vi "ADS1015 Read All.vi"(8 "error in (no error)":errorcluster, 9 "ADS1015 Config Options":T1={"I2C"={"Slave Address"=72, "Channel"=1}, "ADC"={"Channel"=4, "Expected Range (Programmable Gain Amplifier)"=0, "Sampling Mode"=1, "Sampling Rate"=4, "Comparator Mode"=1, "Comparator Polarity"=1, "Latching Comparator"=1, "Comparator Queue & Disable"=3}} {"ADC"."Comparator Queue & Disable" items=["Assert after one conversion", "Assert after two conversions", "Assert after four conversions", "Comparator disabled"]; "ADC"."Latching Comparator" items=["Non-latching", "Latching"]; "ADC"."Comparator Polarity" items=["Active Low", "Active High"]; "ADC"."Comparator Mode" items=["Traditional Comparator w/ hysteresis", "Window Comparator"]; "ADC"."Sampling Rate" items=["128SPS", "250SPS", "490SPS", "920SPS", "1600SPS", "2400SPS", "3300SPS"]; "ADC"."Sampling Mode" items=["Continuous Conversion", "Single-shot (Low Power)"]; "ADC"."Expected Range (Programmable Gain Amplifier)" items=["+/-6.144V", "+/-4.096V", "+/-2.048V", "+/-1.024V", "+/-0.512V", "+/-0.256V"]; "ADC"."Channel" items=["Differential: Ch 0&1", "Differential: Ch 0&3", "Differential: Ch 1&3", "Differential: Ch 2&3", "Single Ended: Ch 0", "Single Ended: Ch 1", "Single Ended: Ch 2", "Single Ended: Ch 3"]; "I2C"."Slave Address" format="%.0x"}, 11 "LINX Resource in":T2) -> (0 "error out":errorcluster, 2 "Voltages":dbl[](array[numeric]) format="%.3f V", 3 "LINX Resource":T2, 4 "Resolutions":dbl[](array[numeric]) format="%.3f V")   [LabVIEW 2017]
uses:
  <vilib>/MakerHub/LINX/Private/Type Defs/Platform.ctl
  <vilib>/MakerHub/LINX/Private/Type Defs/Interface.ctl
  <vilib>/MakerHub/LINX/Private/Device/Type Defs/TCP Config.ctl
  <vilib>/MakerHub/LINX/Private/Device/Type Defs/Channels.ctl
  <vilib>/MakerHub/LINX/Private/Device/Type Defs/LINX Device Config.ctl
  <vilib>/MakerHub/LINX/Private/Type Defs/LINX Ref.ctl
  ADS1015 Config Options.ctl
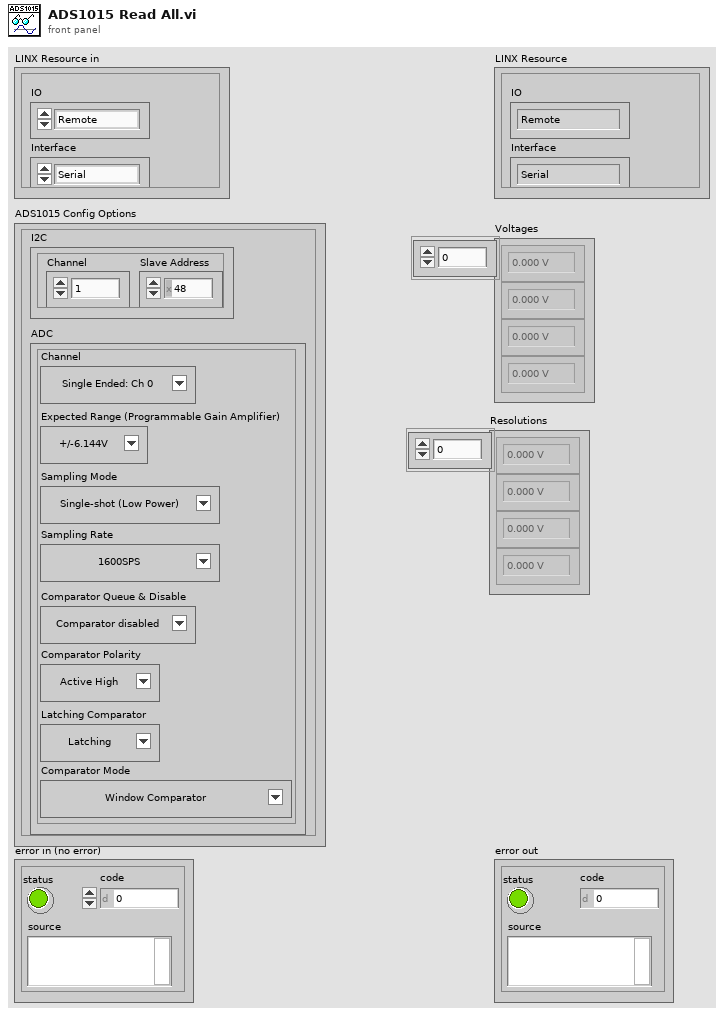
[diagram p1: front panel]
types:
  T1 = typedef "ADS1015 Config Options.ctl" = cluster{"I2C":cluster{"Slave Address":u8, "Channel":u8}, "ADC":cluster{"Channel":u8, "Expected Range (Programmable Gain Amplifier)":u8, "Sampling Mode":u8, "Sampling Rate":u8, "Comparator Mode":u8, "Comparator Polarity":u8, "Latching Comparator":u8, "Comparator Queue & Disable":u8}}
  T2 = typedef "LMH-LINX.lvlib/LINX Ref.ctl" = cluster{"IO":T3, "Interface":T4, "LINX Device Config":T5}
  T3 = typedef "LMH-LINX.lvlib/Platform.ctl" = enum16{"Remote", "Local"}
  T4 = typedef "LMH-LINX.lvlib/Interface.ctl" = enum16{"Serial", "TCP"}
  T5 = typedef "LMH-LINX.lvlib/Device.lvlib/LINX Device Config.ctl" = cluster{"Interface":T4, "COM Port":refnum<visa-resource-name>, "TCP Configuration":T6, "Device Family":u8, "Device ID":u8, "Device Name":string, "TCP Ref":refnum<k5>, "Channels":T7}
  T6 = typedef "LMH-LINX.lvlib/Device.lvlib/TCP Config.ctl" = cluster{"IP Address":string, "Port":u16}
  T7 = typedef "LMH-LINX.lvlib/Channels.ctl" = cluster{"DI":u8[], "DO":u8[], "AI":u8[], "AO":u8[], "PWM":u8[], "QE":u8[], "UART":u8[], "I2C 2":u8[], "SPI":u8[], "CAN":u8[], "Servo":u8[], "AI Ref (V)":dbl, "AI Resolution (Bits)":u8, "AO Ref (V)":dbl, "AO Resolution (Bits)":u8}
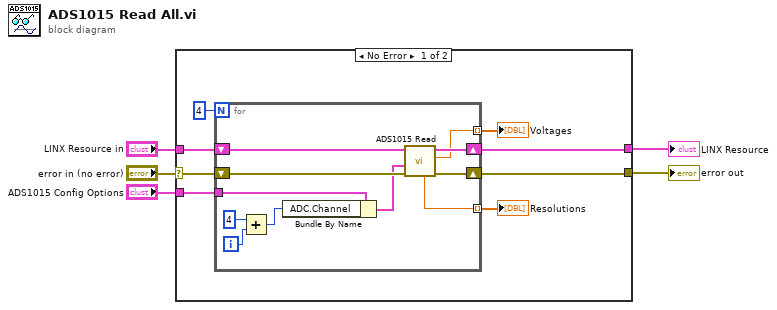
[diagram p0: block diagram]
diagram:
  n1 = case shown="No Error" "error in (no error)" {
    selector: "error in (no error)" -> [w12 w25]
    tunnel: "LINX Resource in" -> [w13 w26]
    tunnel: "ADS1015 Config Options" -> [w11 _]
    tunnel: [w10 w26] -> w2
    tunnel: [w9 w25] -> w1
    frame No Error {
      n2 = for {
        N: 4 -> [_]
        tunnel: w11 -> [w24]
        tunnel: [w15] -> w8 mode=indexing
        shift-right: [w17] -> w10
        shift-left: w13 -> [w20]
        shift-right: [w16] -> w9
        shift-left: w12 -> [w19]
        tunnel: [w14] -> w6 mode=indexing
        i -> [w23]
        n3 = Add(x=4, y=w23) -> (x+y=w21:i32)
        n4 = Bundle By Name(cluster=w24, "ADC.Channel"=w21) -> (w18:T1)
        n5 = call "ADS1015 Read.vi"("error in (no error)"=w19, "ADS1015 Config Options"=w18, "LINX Resource in"=w20) -> ("error out"=w16:errorcluster, "Voltage"=w15:dbl, "LINX Resource"=w17:T2, "Resolution"=w14:dbl)  [unwired: 5 in]
      }
      "Voltages" <- w8
      "Resolutions" <- w6
    }
    frame Error {
    }
  }
  "error out" <- w1
  "LINX Resource" <- w2
